vi "Open.vi"(8 "error in (no error)":errorcluster, 11 "ArgumentParser in":refnum<class "ArgumentParser.lvclass">) -> (0 "error out":errorcluster, 3 "ArgumentParser out":refnum<class "ArgumentParser.lvclass">)   [LabVIEW 2022 SP3, in "ArgumentParser.lvlib" / "ArgumentParser.lvclass"]
uses:
  ArgumentParser.lvclass
  ArgumentParser.lvclass/ArgumentParser.ctl
  ArgparseWrapper/ArgparseWrapper.lvclass
  PathUtils/Source/PathUtils.lvlib
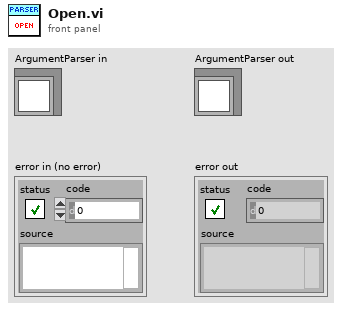
[diagram p1: front panel]
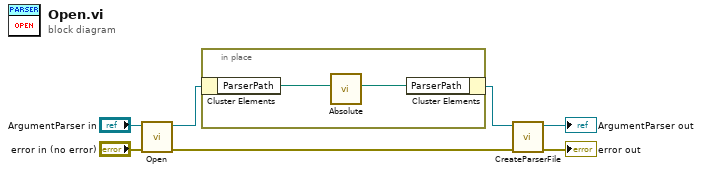
[diagram p0: block diagram]
diagram:
  n1 = call-parent "Open.vi"("error in (no error)"="error in (no error)", "PythonWrapper in"="ArgumentParser in") -> ("error out"=w7:errorcluster, "PythonWrapper out"=w4:refnum<class "ArgumentParser.lvclass">)  [unwired: 8 in]
  n2 = in-place {
    n3 = in-place-cluster #1(w4) -> ("ParserPath"=w9:path)
    n4 = call "Absolute.vi"("Path in"=w9) -> ("Path out"=w8:path)  [unwired: 10 in]
    n5 = in-place-cluster #1("ParserPath"=w8) -> (w2:refnum<class "ArgumentParser.lvclass">)
  }
  n6 = call-dynamic "CreateParserFile.vi"("error in (no error)"=w7, "ArgumentParser in"=w2) -> ("error out"=→"error out":errorcluster, "ArgumentParser out"=→"ArgumentParser out":refnum<class "ArgumentParser.lvclass">)  [unwired: 8 in]
